vi "SetExposure.vi"(1 "Exposure":u32) -> (0 "Error":u32)   [LabVIEW 2012]
uses:
  hidapi_32bits.dll
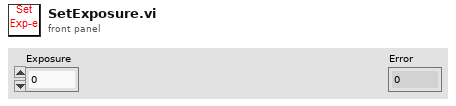
[diagram p1: front panel]
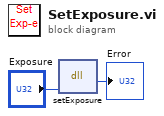
[diagram p0: block diagram]
diagram:
  n1 = dll-call lib="C:/All_Data/mikrocont/Project1/New_controller__Jan_2015/LabView_Aug_2015/hidapi_32bits.dll" fn="setExposure"("Exposure"="Exposure") -> ("Error"=→"Error":u32)  [unwired: 4 in, 2 out]
